vi "EnableDisableControls.vi"(8 "Disabled":T1(ring), 11 "Color indicators ref":refnum<vi>[](array[refnum])) -> ()   [LabVIEW 2019, in "GameLogic.lvlib" / "GameLogic.lvclass"]
uses:
  GameLogic.lvclass
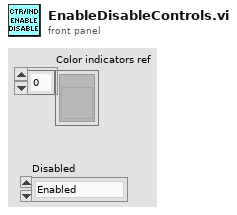
[diagram p1: front panel]
types:
  T1 = enum8{"Enabled", "Disabled", "Disabled and Grayed Out"}
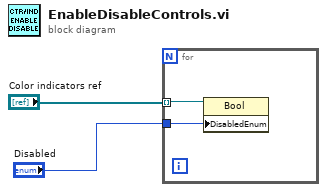
[diagram p0: block diagram]
diagram:
  n1 = for {
    tunnel: "Color indicators ref" -> [w4] mode=indexing
    tunnel: "Disabled" -> [w3]
    n2 = property class="Bool"(reference=w4, "DisabledEnum"=w3) -> ()  [unwired: 1 in, 2 out]
  }
